vi "AutoPickupTote.vi"(10 "Hold Low?":bool) -> (2 "Done?":bool)   [LabVIEW 2014]
uses:
  Rollers/Roller Modes.ctl
  Common Code/Auto Roller Commands.ctl
  Common Code/Roller Mode Enum.ctl
  Elevator/Elevator Command.ctl
  Common Code/Elevator Mode.ctl
  Common Code/Change Detect Int.vi
  Robot Global Data.vi
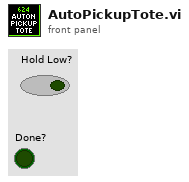
[diagram p1: front panel]
types:
  T1 = typedef "Roller Modes.ctl" = cluster{"Auto Roller Command":T2, "Roller Mode":T3, "Override Intake Speed":dbl}
  T2 = typedef "Auto Roller Commands.ctl" = enum16{"Drag Tote", "Grab Tote", "Idle", "Eject Tote", "Untip Can", "Grab Can"}
  T3 = typedef "Roller Mode Enum.ctl" = enum16{"Manual", "Safe", "Auto"}
  T4 = typedef "Elevator Mode.ctl" = enum16{"Manual", "Safe", "Auto"}
  T5 = typedef "Elevator Command.ctl" = enum16{"Idle", "Load 1", "Load 2", "Load 3", "Drop Stack", "Eject Stack", "Untip Trashcan", "Load Trashcan", "HP Load", "HP Score"}
  T6 = typedef "Elevator Control Command.ctl" = cluster{"Command":T5, "Manual Motor Out":dbl, "Manual Eject Piston":bool, "Mode":T4, "Override Limits":bool, "Manual Stabilizer":bool, "Manual Finger":bool, "Store Trashcan?":bool, "Hold Low?":bool, "Idle Mode":T7, "HP Load":bool, "Unstick":bool}
  T7 = typedef "Elevator Idle Mode.ctl" = enum16{"Load 1", "Load 2", "Load 3", "Load Can", "Untip Can", "Step Load", "Drop Stack"}
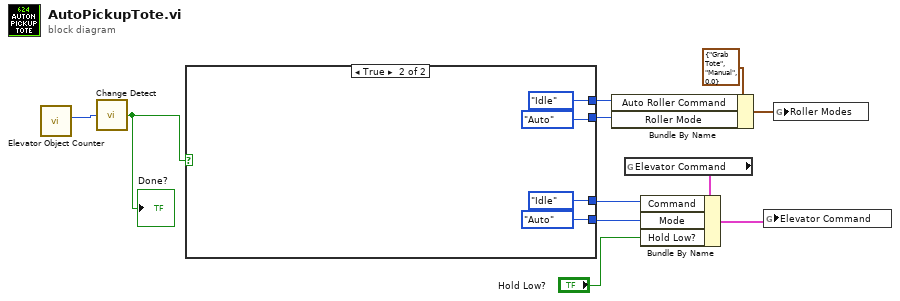
[diagram p0: block diagram]
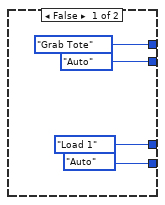
[diagram p2: hidden frame]
diagram:
  n1 = call "Elevator Object Counter.vi"() -> ("Tote Count"=w8:i8)  [unwired: 10 in, 1 out]
  n2 = call-poly "Change Detect.vi"("In"=w8) -> ("Changed?"=w7:bool)
  "Done?" <- w7
  n3 = case shown="True" w7 {
    tunnel: [Auto_Roller_Commands."Grab Tote" ("Auto Roller Command") Auto_Roller_Commands."Idle" ("Auto Roller Command")] -> w6
    tunnel: [Roller_Mode_Enum."Auto" ("Roller Mode") Roller_Mode_Enum."Auto" ("Roller Mode")] -> w5
    tunnel: [Elevator_Command."Load 1" ("Command") Elevator_Command."Idle" ("Command")] -> w4
    tunnel: [Elevator_Mode."Auto" ("Mode") Elevator_Mode."Auto" ("Mode")] -> w3
    frame False {
    }
    frame True {
    }
  }
  n4 = Bundle By Name(cluster=T1 {"Auto Roller Command"=enum."Grab Tote", "Roller Mode"=enum."Manual", "Override Intake Speed"=0.0} ("Roller Modes"), "Auto Roller Command"=w6, "Roller Mode"=w5) -> (w9:T1)
  n5 = global read "Robot Global Data.vi" "Elevator Command"() -> (w1:T6)
  n6 = Bundle By Name(cluster=w1, "Command"=w4, "Mode"=w3, "Hold Low?"="Hold Low?") -> (w11:T6)
  n7 = global write "Robot Global Data.vi" "Elevator Command"(w11) -> ()
  n8 = global write "Robot Global Data.vi" "Roller Modes"(w9) -> ()
